vi "Configuration Tool Main.vi"() -> ()   [LabVIEW 2015, in "Configuration Tool.lvlib"]
doc: "This is the main VI for the configuration editor."
uses:
  Configuration Tool.lvlib
  Controls/StateCluster.ctl
  <vilib>/NI/Configuration Framework/Repository/NISE_CEF_Repository.lvclass
  <vilib>/NI/Configuration Framework/Node/NodeRef.ctl
  <vilib>/NI/Configuration Framework/Node/NISE_CEF_Node.lvclass
  <vilib>/NI/Configuration Framework/Node/StandardEvents.ctl
  <vilib>/NI/Configuration Framework/Node/UserEventRef.ctl
  <vilib>/NI/Configuration Framework/Controls/EventCluster.ctl
  <vilib>/NI/Configuration Framework/Node/NodeChangeEvent.ctl
  <vilib>/NI/Configuration Framework/Node/CacheState.ctl
  <vilib>/NI/Configuration Framework/Node/RefreshUIEvent.ctl
  <vilib>/NI/Configuration Framework/Node/StopEvent.ctl
  <vilib>/NI/Configuration Framework/glyph manager/glyph manager.ctl
  <vilib>/picture/picture.llb/imagedata.ctl
  Controls/AddMessage.ctl
  Controls/MoveMessage.ctl
  <vilib>/Utility/error.llb/DialogType.ctl
  Classes/Custom Device/CustomDevice.lvclass
  Classes/CustomDeviceRepo/CustomDeviceRepo.lvclass
  <vilib>/Utility/sysdir.llb/System Directory Type.ctl
  <vilib>/NI/AMC/Read Termination Message.vi
  <vilib>/NI/AMC/Create Single Message.vi
  <vilib>/NI/AMC/Update Message Routing Info.vi
  subVI/Global Settings.vi
  <vilib>/NI/AMC/Globals.vi
  <vilib>/NI/AMC/Send Message.vi
  <vilib>/NI/AMC/AMC.lvlib
  <vilib>/NI/Configuration Framework/NISE_CEF_TreeControl.lvlib
  <vilib>/NI/Configuration Framework/glyph manager/glyph manager.lvlib
panel:
  in  "Target Project":string(combo)
  in  "VeriStand Version":enum16{"2013", "2014", "2015", "2016"}(ring)=enum."2015"
  in  "View":string(tree)
  in  "Exit":bool
  # "Custom Device XML Editor"
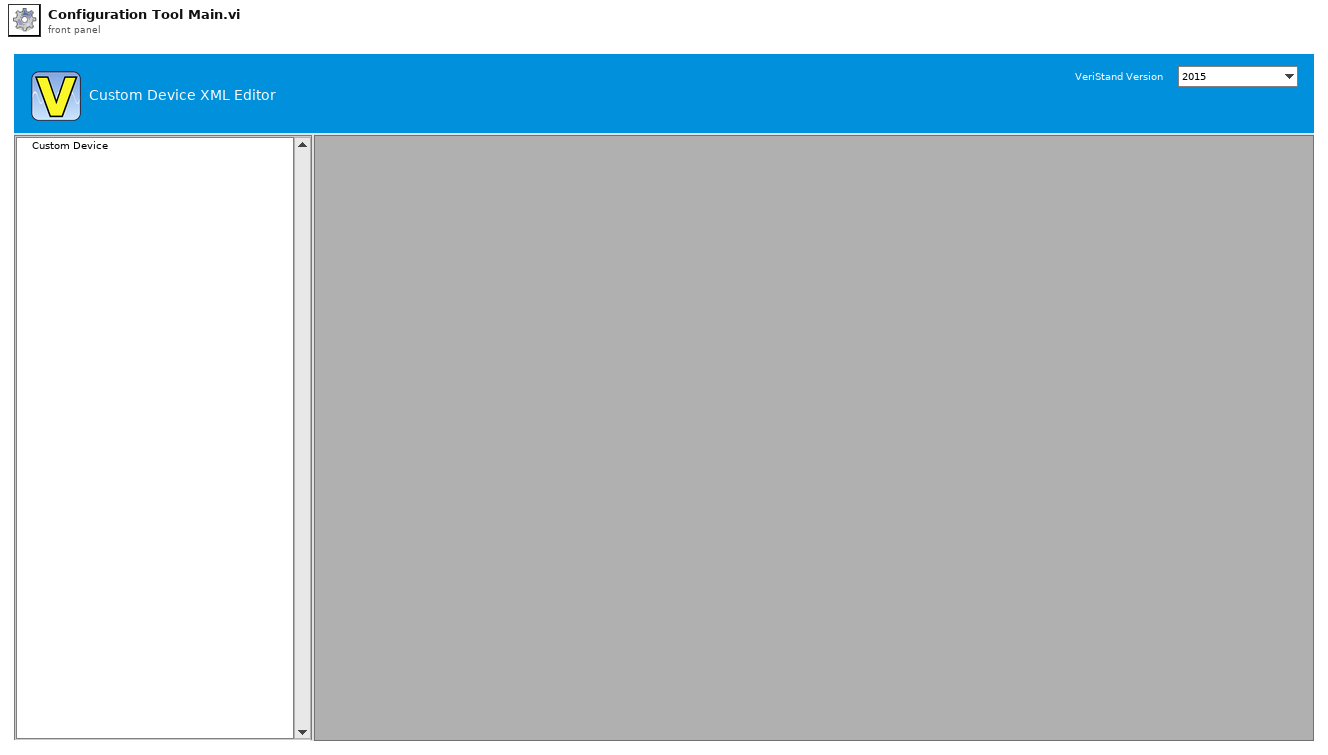
[diagram p1: front panel]
types:
  T1 = typedef "Configuration Tool.lvlib/StateCluster.ctl" = cluster{"repository":refnum<class "NISE_CEF_Repository.lvclass">, "root":T2, "unsaved changes":bool, "current path":path, "standard events":T3, "classes path":path, "glyph manager":T9}
  T2 = typedef "NISE_CEF_Node.lvclass/NodeRef.ctl" = refnum<data-value>
  T3 = typedef "NISE_CEF_Node.lvclass/StandardEvents.ctl" = cluster{"user event":T4, "node change":T5, "cache state":T6, "refresh UI":T7, "stop event":T8}
  T4 = typedef "NISE_CEF_Node.lvclass/UserEventRef.ctl" = refnum<user-event>
  T5 = typedef "NISE_CEF_Node.lvclass/NodeChangeEvent.ctl" = refnum<user-event>
  T6 = typedef "NISE_CEF_Node.lvclass/CacheState.ctl" = refnum<user-event>
  T7 = typedef "NISE_CEF_Node.lvclass/RefreshUIEvent.ctl" = refnum<user-event>
  T8 = typedef "NISE_CEF_Node.lvclass/StopEvent.ctl" = refnum<user-event>
  T9 = typedef "glyph manager.lvlib/glyph manager.ctl" = cluster{"search paths":path[], "glyph map":variant, "base glyphs":T10[], "desired overlays":string[]}
  T10 = typedef "imagedata.ctl" = cluster{"image type":i32, "image depth":i32, "image":u8[], "mask":u8[], "colors":u32[], "Rectangle":cluster{"left":i16, "top":i16, "right":i16, "bottom":i16}}
  T11 = cluster{"Names":string[], "Project refs":refnum<vi>[]}
  T12 = typedef "AMC.lvlib/Message Queue.ctl" = refnum<queue>
  T13 = typedef "Configuration Tool.lvlib/AddMessage.ctl" = cluster{"node type":string, "to add to":string}
  T14 = typedef "Configuration Tool.lvlib/MoveMessage.ctl" = cluster{"node ref":T2, "new parent":T2}
  T15 = typedef "Configuration Tool.lvlib/FilePaths.ctl" = cluster{"glyphs":path, "classes":path}
  T16 = typedef "DialogType.ctl" = u16
  T17 = typedef "System Directory Type.ctl" = i32
  T18 = typedef "NISE_CEF_Node.lvclass/Summary.ctl" = cluster{"ID":string, "parent ID":string, "node type":string, "text":string, "additional text":string, "glyph":string, "depth":i32, "glyph overlay":string}
  T19 = typedef "LVPoint32TypeDef.ctl" = cluster{"Horizontal":i32, "Vertical":i32}
  T20 = cluster{"data name":string, "drag data":variant}[]
  T21 = typedef "NISE_CEF_Node.lvclass/NodeMenuOptions.ctl" = cluster{"removable":bool, "movable":bool, "duplicate":bool}
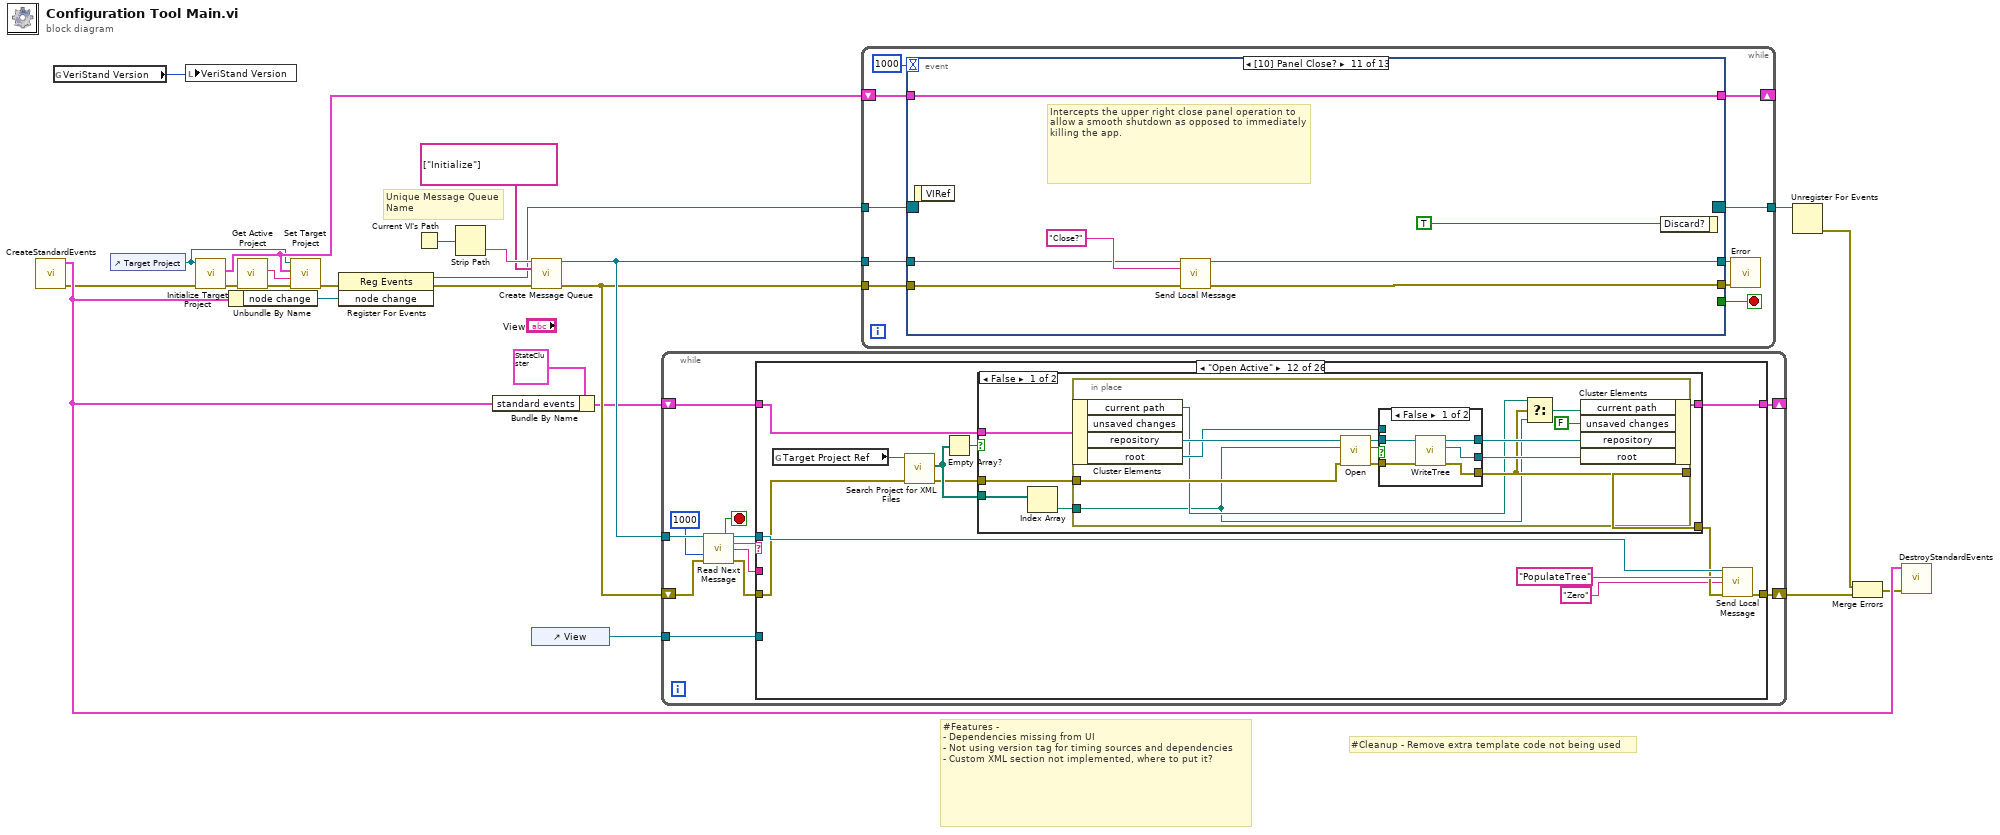
[diagram p0: block diagram]
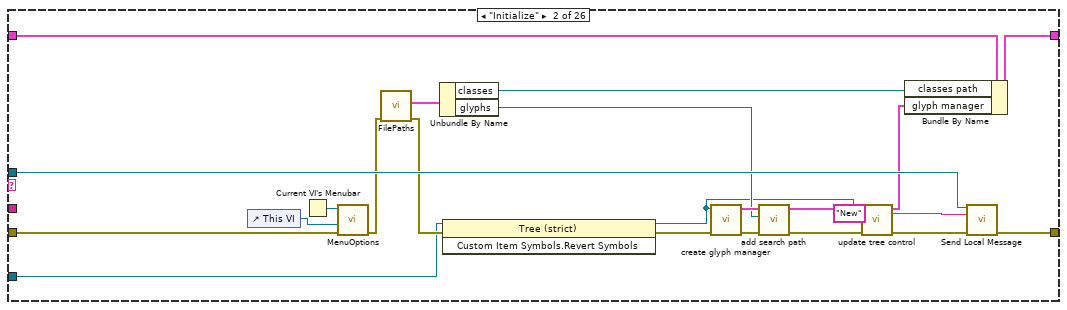
[diagram p3: hidden frame]
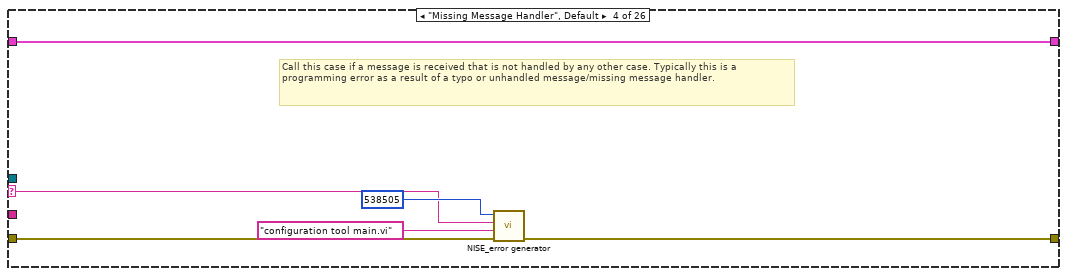
[diagram p5: hidden frame]
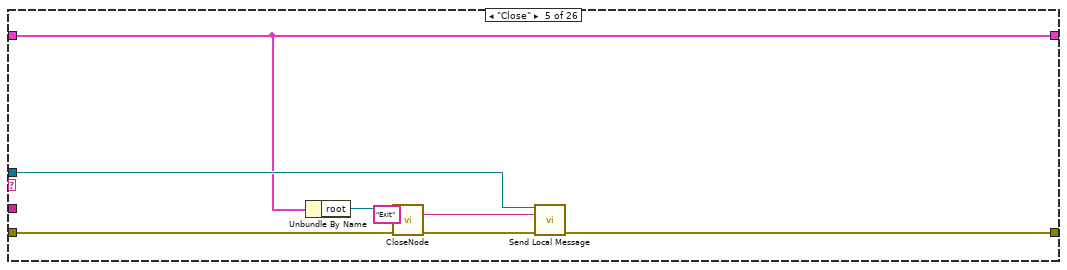
[diagram p6: hidden frame]
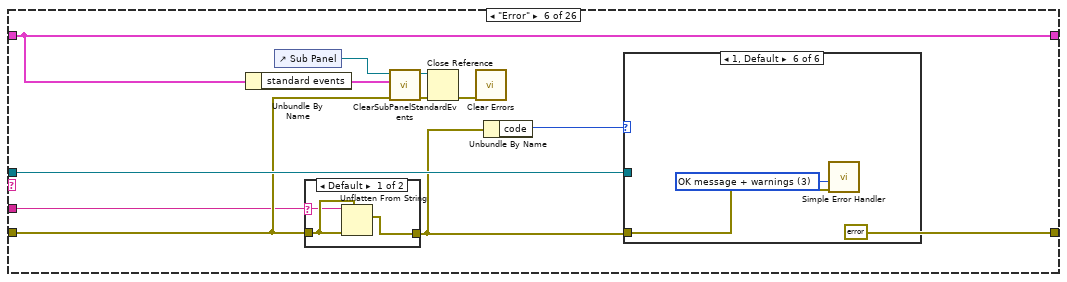
[diagram p7: hidden frame]
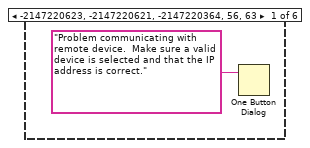
[diagram p9: hidden frame]
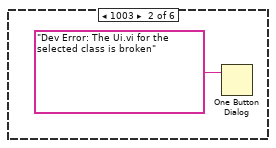
[diagram p10: hidden frame]
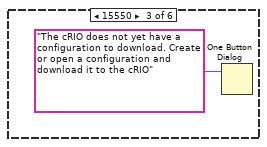
[diagram p11: hidden frame]
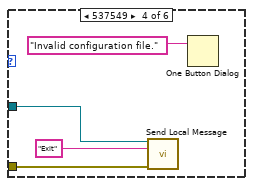
[diagram p12: hidden frame]
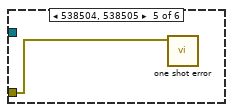
[diagram p13: hidden frame]
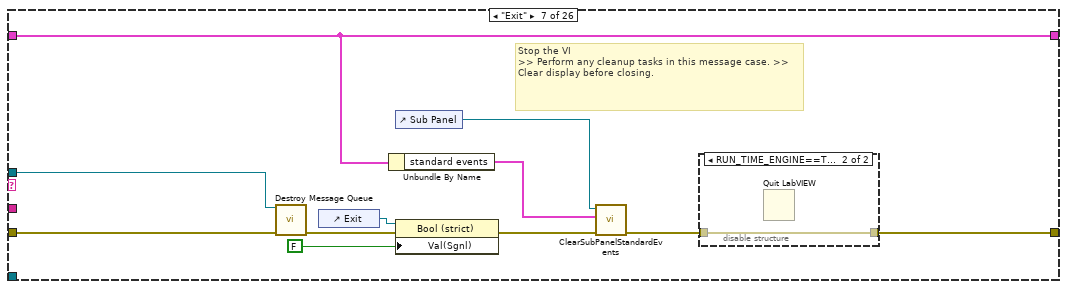
[diagram p14: hidden frame]
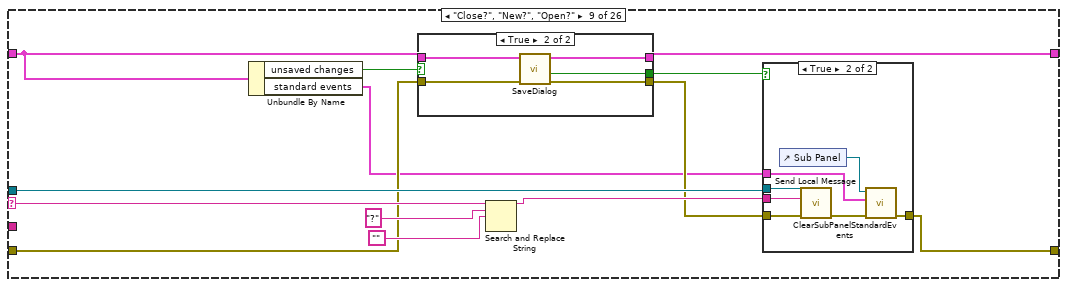
[diagram p17: hidden frame]
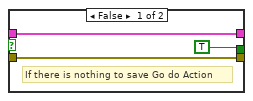
[diagram p18: hidden frame]
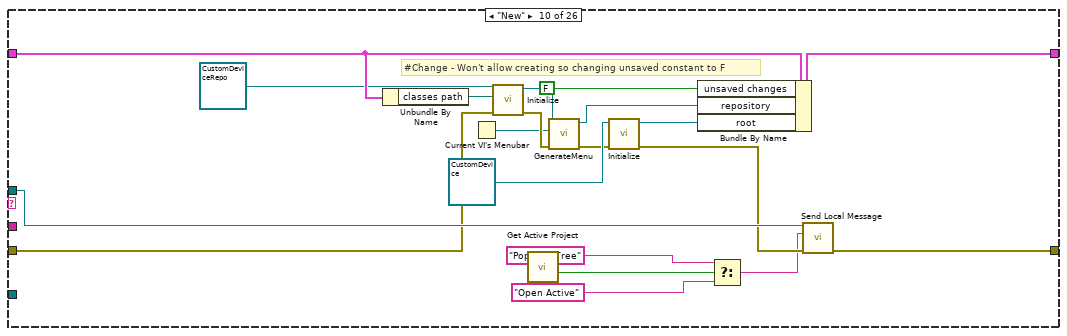
[diagram p20: hidden frame]
diagram:
  # "#Cleanup - Remove extra template code not being used"
  # "#Features - \n- Dependencies missing from UI\n- Not using version tag for timing sources and dependencies\n- Custom XML section not implemented, where to put it?"
  # "Unique Message Queue Name"
  n1 = call <vilib>:"CreateStandardEvents.vi"() -> ("error out"=w2:errorcluster, "standard events"=w14:T3)  [unwired: 10 in]
  n2 = global read "Global Settings.vi" "VeriStand Version"() -> (w8:enum16{"2013", "2014", "2015", "2016"})
  n3 = control-ref of="Target Project"() -> (w3:refnum<vi>)
  n4 = local write "VeriStand Version"(w8) -> ()
  n5 = call "Initialize Target Project.vi"("error in (no error)"=w2, "ComboBox in"=w3) -> ("error out"=w7:errorcluster, "Projects"=w5:T11)  [unwired: 8 in]
  n6 = Unbundle By Name(w14) -> ("node change"=w19:T5)
  n7 = call "Get Active Project.vi"("error in (no error)"=w7) -> ("error out"=w6:errorcluster, "Name"=w4:string)  [unwired: 7 in, 2 out]
  n8 = call "Set Target Project.vi"("error in (no error)"=w6, "Target Project"=w4, "Projects"=w5, "ComboBox Ref"=w3) -> ("error out"=w1:errorcluster)  [unwired: 7 in]
  n9 = register-events(error in=w1, w19) -> (reference out=w13:refnum<event-registration>, error out=w18:errorcluster)  [unwired: 1 in]
  n10 = Current VI's Path() -> (path=w23:path)
  n11 = Strip Path(path=w23) -> (name=w24:string)  [unwired: 1 out]
  n12 = Bundle By Name(cluster=T1 {"repository"=refnum, "root"=refnum, "unsaved changes"=FALSE, "current path"=path "", "standard events"={"user event"=refnum, "node change"=refnum, "cache state"=refnum, "refresh UI"=refnum, "stop event"=refnum}, "classes path"=path "", "glyph manager"={"search paths"=[], "glyph map"=variant, "base glyphs"=[], "desired overlays"=[]}}, "standard events"=w14) -> (w16:T1)
  n13 = call <vilib>:"Create Message Queue.vi"("message queue name"=w24, "initial message names"=string[] ["Initialize"], "error in"=w18) -> ("message queue out"=w21:T12, "error out"=w20:errorcluster)  [unwired: 11 in]
  n14 = control-ref of="View"() -> (w12:refnum<vi>)
  n15 = while "Message Processor" {
    shift-right: [w32] -> w15
    shift-left: w20 -> [w31]
    tunnel: w21 -> [w30]
    shift-right: [w28] -> _
    shift-left: w16 -> [w27]
    tunnel: w12 -> [w25]
    stop <- w36 stop-if-true
    n16 = call <vilib>:"Read Next Message.vi"("message queue in"=w30, "timeout (1 ms)"=1000, "error in"=w31) -> ("exit process?"=w36:bool, "message queue out"=w26:T12, "message name"=w35:string, "message value"=w34:string, "error out"=w33:errorcluster)  [unwired: 5 in, 3 out]
    n17 = case shown="\"Open Active\"" w35 {
      selector: w35 -> [_ _ _ w64 _ _ _ _ w125 _ _ _ _ _ _ _ _ _ w382 _ _ _ _ _ _ _]
      tunnel: w34 -> [_ _ _ _ _ w77 _ _ _ _ _ _ _ _ w291 _ w343 w360 w380 w432 w456 w467 _ w516 w536 w543]
      tunnel: w33 -> [w38 w60 w62 w67 w70 w80 w112 w116 w118 w159 w179 w218 w261 w283 w298 w311 w336 w359 w385 w434 w455 w484 w506 w515 w534 w544]
      tunnel: [w38 w56 w62 w65 w74 errorcluster {"status"=FALSE, "code"=0, "source"=""} ("error out") w104 w116 w129 w165 w175 w223 w258 w285 w295 w311 w315 w363 w388 w436 w452 w471 w502 w512 w529 w542] -> w32
      tunnel: [w37 w52 w61 w68 w72 w84 w103 w115 w120 w163 w180 w227 w264 w284 w292 w310 w331 w356 w389 w435 w457 w477 w505 w510 w537 w539] -> w28
      tunnel: w27 -> [w37 w53 w61 w68 w72 w84 w103 w115 w121 w161 w181 w228 w263 w282 w293 w310 w334 w357 w389 w427 w457 w486 w505 w510 w537 w545]
      tunnel: w26 -> [_ w55 _ _ w73 w87 w111 _ w128 w164 w177 w225 _ _ w294 _ w312 _ w383 _ _ _ _ w511 w528 w541]
      tunnel: w25 -> [_ w41 _ _ _ _ _ _ _ _ _ _ _ _ _ _ w332 w352 w377 w429 w450 w473 _ _ _ _]
      frame "------------Generic Operations------------" {
        # "Dummy case to add a seperation in the Case Structure menu"
      }
      frame "Initialize" {
        n18 = control-ref of="This VI"() -> (w59:refnum<vi>)
        n19 = Current VI's Menubar() -> (w58:refnum<k9>)
        n20 = call "MenuOptions.vi"("error in"=w60, "VI ref"=w59, "menu ref in"=w58) -> ("error out"=w51:errorcluster)  [unwired: 7 in, 1 out]
        n21 = call "FilePaths.vi"("error in"=w51) -> ("error out"=w44:errorcluster, "paths"=w54:T15)  [unwired: 9 in]
        n22 = Unbundle By Name(w54) -> ("classes"=w50:path, "glyphs"=w46:path)
        n23 = invoke class="Tree (strict)" method="Custom Item Symbols.Revert Symbols"(reference=w41, error in=w44) -> (reference out=w42:refnum<vi>, error out=w43:errorcluster)  [unwired: 1 in, 1 out]
        n24 = call <vilib>:"create glyph manager.vi"("error in"=w43, "tree ref (for default symbols)"=w42) -> ("error out"=w49:errorcluster, "glyph manager"=w48:T9)  [unwired: 8 in]
        n25 = call <vilib>:"add search path.vi"("error in"=w49, "search path"=w46, "glyph manager in"=w48) -> ("error out"=w40:errorcluster, "glyph manager out"=w39:T9)  [unwired: 7 in]
        n26 = call <vilib>:"update tree control.vi"("error in"=w40, "tree reference"=w42, "glyph manager in"=w39) -> ("error out"=w47:errorcluster, "glyph manager out"=w45:T9)  [unwired: 7 in]
        n27 = Bundle By Name(cluster=w53, "classes path"=w50, "glyph manager"=w45) -> (w52:T1)
        n28 = call <vilib>:"Send Local Message.vi"("message queue in"=w55, "message name"="New" ("Message Name"), "error in"=w47) -> ("error out"=w56:errorcluster)  [unwired: 10 in, 2 out]
      }
      frame "", "Idle" {
      }
      frame "Missing Message Handler", Default {
        # "Call this case if a message is received that is not handled by any other case. Typically this is a programming error as a result of a typo or unhandled message/missing message handler."
        n29 = call <vilib>:"NISE_error generator.vi"("error in"=w67, "source"="configuration tool main.vi", "append error message"=w64, "error code (0)"=538505) -> ("error out"=w65:errorcluster)  [unwired: 5 in]
      }
      frame "Close" {
        n30 = Unbundle By Name(w72) -> ("root"=w71:T2)
        n31 = call <vilib>:"CloseNode.vi"("error in"=w70, "node ref"=w71) -> ("error out"=w69:errorcluster)  [unwired: 9 in]
        n32 = call <vilib>:"Send Local Message.vi"("message queue in"=w73, "message name"="Exit", "error in"=w69) -> ("error out"=w74:errorcluster)  [unwired: 10 in, 2 out]
      }
      frame "Error" {
        n33 = Unbundle By Name(w84) -> ("standard events"=w76:T3)
        n34 = control-ref of="Sub Panel"() -> (w83:refnum<vi>)
        n35 = case shown="Default" w77 {
          selector: w77 -> [w89 _]
          tunnel: w80 -> [w90 w91]
          tunnel: [w88 w91] -> w79
          frame Default {
            n36 = Unflatten From String(type=w90, binary string=w89, error in (no error)=w90) -> (value=w88:errorcluster)  [unwired: 2 in, 2 out]
          }
          frame "" {
          }
        }
        n37 = call <vilib>:"ClearSubPanelStandardEvents.vi"("error in"=w80, "standard events"=w76, "sub panel ref in"=w83) -> ("error out"=w82:errorcluster, "sub panel ref out"=w81:refnum<vi>)  [unwired: 7 in]
        n38 = Close Reference(reference=w81, error in (no error)=w82) -> (error out=w78:errorcluster)
        n39 = call <vilib>:"Clear Errors.vi"("error in (no error)"=w78) -> ()  [unwired: 5 in, 2 out]
        n40 = Unbundle By Name(w79) -> ("code"=w85:i32)
        n41 = case shown="1, Default" w85 {
          tunnel: w87 -> [_ _ _ w97 _ _]
          tunnel: w79 -> [_ _ _ w96 w99 w101]
          frame -2147220623, -2147220621, -2147220364, 56, 63 {
            n42 = One Button Dialog(message="Problem communicating with remote device.  Make sure a valid device is selected and that the IP address is correct.") -> ()  [unwired: 1 in, 1 out]
          }
          frame 1003 {
            n43 = One Button Dialog(message="Dev Error: The Ui.vi for the selected class is broken") -> ()  [unwired: 1 in, 1 out]
          }
          frame 15550 {
            n44 = One Button Dialog(message="The cRIO does not yet have a configuration to download. Create or open a configuration and download it to the cRIO") -> ()  [unwired: 1 in, 1 out]
          }
          frame 537549 {
            n45 = call <vilib>:"Send Local Message.vi"("message queue in"=w97, "message name"="Exit", "error in"=w96) -> ()  [unwired: 10 in, 3 out]
            n46 = One Button Dialog(message="Invalid configuration file.") -> ()  [unwired: 1 in, 1 out]
          }
          frame 538504, 538505 {
            n47 = call <vilib>:"one shot error.vi"("error in"=w99) -> ()  [unwired: 11 in]
          }
          frame 1, Default {
            w100 = T16 3 items=["no dialog", "OK message", "continue or stop message", "OK message + warnings", "continue/stop + warnings"] ("type of dialog (OK msg:1)")
            n48 = call <vilib>:"Simple Error Handler.vi"("type of dialog (OK msg:1)"=w100, "error in (no error)"=w101) -> ()  [unwired: 8 out]
          }
        }
      }
      frame "Exit" {
        # "Stop the VI                                                                             >> Perform any cleanup tasks in this message case. >> Clear display before closing."
        n49 = call <vilib>:"Destroy Message Queue.vi"("message queue in"=w111, "error in"=w112) -> ("error out"=w108:errorcluster)  [unwired: 11 in, 2 out]
        n50 = control-ref of="Exit"() -> (w110:refnum<vi>)
        n51 = Unbundle By Name(w103) -> ("standard events"=w102:T3)
        n52 = control-ref of="Sub Panel"() -> (w107:refnum<vi>)
        n53 = property class="Bool (strict)"(reference=w110, error in=w108, "Val(Sgnl)"=FALSE ("Exit")) -> (error out=w106:errorcluster)  [unwired: 1 out]
        n54 = call <vilib>:"ClearSubPanelStandardEvents.vi"("error in"=w106, "standard events"=w102, "sub panel ref in"=w107) -> ("error out"=w105:errorcluster)  [unwired: 7 in, 1 out]
        n55 = disable-structure shown="RUN_TIME_ENGINE==True" {
          disable-tunnel: [w113 w114] -> w104
          disable-tunnel: w105 -> [w113 w114]
          frame condition #0 (active) {
          }
          frame condition #1 {
            n56 = Quit LabVIEW() -> ()  [unwired: 1 in]
          }
        }
      }
      frame "------------Menu Operations--------------" {
        # "Dummy case to add a seperation in the Case Structure menu"
      }
      frame "Close?", "New?", "Open?" {
        n57 = Unbundle By Name(w121) -> ("unsaved changes"=w123:bool, "standard events"=w117:T3)
        n58 = case shown="True" w123 {
          tunnel: [TRUE ("SaveFlag") w137] -> w122
          tunnel: w121 -> [w131 w136]
          tunnel: [w131 w135] -> w120
          tunnel: w118 -> [w130 w134]
          tunnel: [w130 w133] -> w119
          frame False {
            # "If there is nothing to save Go do Action"
          }
          frame True {
            n59 = call "SaveDialog.vi"("error in"=w134, "state in"=w136) -> ("error out"=w133:errorcluster, "new"=w137:bool, "state out"=w135:T1)  [unwired: 7 in]
          }
        }
        n60 = Search and Replace String(input string=w125, search string="?", replace string="") -> (result string=w124:string)  [unwired: 5 in, 3 out]
        n61 = case shown="True" w122 {
          tunnel: w119 -> [w138 w145]
          tunnel: [w138 w141] -> w129
          tunnel: w128 -> [_ w144]
          tunnel: w124 -> [_ w143]
          tunnel: w117 -> [_ w139]
          frame False {
          }
          frame True {
            n62 = control-ref of="Sub Panel"() -> (w140:refnum<vi>)
            n63 = call <vilib>:"Send Local Message.vi"("message queue in"=w144, "message name"=w143, "error in"=w145) -> ("error out"=w142:errorcluster)  [unwired: 10 in, 2 out]
            n64 = call <vilib>:"ClearSubPanelStandardEvents.vi"("error in"=w142, "standard events"=w139, "sub panel ref in"=w140) -> ("error out"=w141:errorcluster)  [unwired: 7 in, 1 out]
          }
        }
      }
      frame "New" {
        # "#Change - Won't allow creating so changing unsaved constant to F"
        n65 = Unbundle By Name(w161) -> ("classes path"=w160:path)
        n66 = Current VI's Menubar() -> (w155:refnum<k9>)
        n67 = call-dynamic "Initialize.vi"("error in"=w159, "path"=w160, "repository in"=refnum<class "CustomDeviceRepo.lvclass"> refnum ("CustomDeviceRepo.lvclass")) -> ("error out"=w158:errorcluster, "repository out"=w157:refnum<class "CustomDeviceRepo.lvclass">)  [unwired: 7 in]
        n68 = call "Get Active Project.vi"() -> ("No Active Project?"=w149:bool)  [unwired: 8 in, 3 out]
        n69 = call-dynamic "GenerateMenu.vi"("error in"=w158, "menu ref in"=w155, "NISE_CEF_Repository in"=w157) -> ("error out"=w152:errorcluster, "NISE_CEF_Repository out"=w156:refnum<class "CustomDeviceRepo.lvclass">)  [unwired: 6 in, 1 out]
        n70 = call-dynamic "Initialize.vi"("error in"=w152, "node in"=refnum<class "CustomDevice.lvclass"> refnum ("CustomDevice.lvclass")) -> ("error out"=w151:errorcluster, "data value reference"=w154:T2)  [unwired: 7 in, 1 out]
        n71 = Bundle By Name(cluster=w161, "unsaved changes"=FALSE ("SaveFlag"), "repository"=w156, "root"=w154) -> (w163:T1)
        n72 = Select(t="PopulateTree", s=w149, f="Open Active") -> (s? t:f=w146:string)
        n73 = call <vilib>:"Send Local Message.vi"("message queue in"=w164, "message name"=w146, "error in"=w151) -> ("error out"=w165:errorcluster)  [unwired: 10 in, 2 out]
      }
      frame "Open" {
        w174 = T17 6 items=["User Home"=0, "User Desktop"=1, "User Documents"=2, "User Application Data"=3, "User Preferences"=4, "User Temporary"=5, "Public Documents"=6, "Public Application Data"=7, "Public Preferences"=8, "Public Cache"=13, "System Core Libraries"=9, "System Installed Libraries"=10, "Application Files"=11, "Boot Volume Root"=12] ("system directory type")
        n74 = global read "Global Settings.vi" "VeriStand Version"() -> (w167:enum16{"2013", "2014", "2015", "2016"})
        n75 = Format Into String(w167) -> (resulting string=w166:string)  [unwired: 3 in, 1 out]
        n76 = Search and Replace String(input string="National Instruments\\NI VeriStand XXXX\\Custom Devices", search string="XXXX", replace string=w166) -> (result string=w170:string)  [unwired: 5 in, 3 out]
        n77 = call <vilib>:"Get System Directory.vi"("system directory type"=w174) -> ("system directory"=w171:path)  [unwired: 10 in]
        n78 = Build Path(base path=w171, name or relative path=w170) -> (appended path=w169:path)
        n79 = in-place {
          in-place-border: w179 -> [w187]
          in-place-border: [w186] -> w176
          in-place-border: w169 -> [w182]
          n80 = in-place-cluster #1(w181) -> ("current path"=w184:path, "repository"=w195:refnum<class "NISE_CEF_Repository.lvclass">, "root"=w191:T2)  [unwired: 1 out]
          n81 = call "FileDialog.vi"("error in"=w187, "start path"=w182) -> ("error out"=w188:errorcluster, "cancelled"=w189:bool, "selected path"=w185:path)  [unwired: 7 in]
          n82 = Compound Arithmetic op=OR(invert w189) -> (w190:bool)
          n83 = case shown="True" w190 {
            tunnel: w195 -> [w196 w208]
            tunnel: [w196 w206] -> w193
            tunnel: [w197 w204] -> w186
            tunnel: [w198 w203] -> w192
            tunnel: w185 -> [_ w201]
            tunnel: w188 -> [w197 w200]
            tunnel: w191 -> [w198 w199]
            frame False {
            }
            frame True {
              n84 = call-dynamic "Open.vi"("error in"=w200, "file path"=w201, "repository in"=w208) -> ("error out"=w205:errorcluster, "invalid?"=w202:bool, "repository out"=w207:refnum<class "NISE_CEF_Repository.lvclass">)  [unwired: 6 in]
              n85 = case shown="False" w202 {
                tunnel: w207 -> [w213 w216]
                tunnel: [w212 w216] -> w206
                tunnel: w205 -> [w211 w215]
                tunnel: [w210 w215] -> w204
                tunnel: [w209 w214] -> w203
                tunnel: w199 -> [_ w214]
                frame False {
                  n86 = call-dynamic "WriteTree.vi"("error in"=w211, "repository in"=w213) -> ("error out"=w210:errorcluster, "root"=w209:T2, "repository out"=w212:refnum<class "NISE_CEF_Repository.lvclass">)  [unwired: 7 in]
                }
                frame True {
                }
              }
            }
          }
          n87 = Select(t=w184, s=w186, f=w185) -> (s? t:f=w183:path)
          n88 = in-place-cluster #1("current path"=w183, "unsaved changes"=FALSE ("SaveFlag"), "repository"=w193, "root"=w192) -> (w180:T1)
        }
        n89 = call <vilib>:"Send Local Message.vi"("message queue in"=w177, "message name"="PopulateTree", "message value"="Zero", "error in"=w176) -> ("error out"=w175:errorcluster)  [unwired: 9 in, 2 out]
      }
      frame "Open Active" {
        n90 = global read "Global Settings.vi" "Target Project Ref"() -> (w221:refnum<vi>)
        n91 = call "Search Project for XML Files.vi"("error in (no error)"=w218, "project reference"=w221) -> ("error out"=w217:errorcluster, "xml files found"=w220:path[])  [unwired: 8 in]
        n92 = Empty Array?(array=w220) -> (empty?=w219:bool)
        n93 = case shown="False" w219 {
          tunnel: w228 -> [w234 w257]
          tunnel: [w233 w257] -> w227
          tunnel: w217 -> [w232 w256]
          tunnel: [w231 w256] -> w224
          tunnel: w220 -> [w229 _]
          frame False {
            n94 = Index Array(array=w229) -> (element=w230:path)  [unwired: 1 in]
            n95 = in-place {
              in-place-border: w232 -> [w242]
              in-place-border: [w241] -> w231
              in-place-border: w230 -> [w235]
              n96 = in-place-cluster #2(w234) -> ("current path"=w240:path, "repository"=w247:refnum<class "NISE_CEF_Repository.lvclass">, "root"=w243:T2)  [unwired: 1 out]
              n97 = call-dynamic "Open.vi"("error in"=w242, "file path"=w235, "repository in"=w247) -> ("error out"=w237:errorcluster, "invalid?"=w236:bool, "repository out"=w238:refnum<class "NISE_CEF_Repository.lvclass">)  [unwired: 6 in]
              n98 = case shown="False" w236 {
                tunnel: w238 -> [w252 w255]
                tunnel: [w251 w255] -> w245
                tunnel: w237 -> [w250 w254]
                tunnel: [w249 w254] -> w241
                tunnel: [w248 w253] -> w244
                tunnel: w243 -> [_ w253]
                frame False {
                  n99 = call-dynamic "WriteTree.vi"("error in"=w250, "repository in"=w252) -> ("error out"=w249:errorcluster, "root"=w248:T2, "repository out"=w251:refnum<class "NISE_CEF_Repository.lvclass">)  [unwired: 7 in]
                }
                frame True {
                }
              }
              n100 = Select(t=w240, s=w241, f=w235) -> (s? t:f=w239:path)
              n101 = in-place-cluster #2("current path"=w239, "unsaved changes"=FALSE ("SaveFlag"), "repository"=w245, "root"=w244) -> (w233:T1)
            }
          }
          frame True {
          }
        }
        n102 = call <vilib>:"Send Local Message.vi"("message queue in"=w225, "message name"="PopulateTree", "message value"="Zero", "error in"=w224) -> ("error out"=w223:errorcluster)  [unwired: 9 in, 2 out]
      }
      frame "Save" {
        n103 = in-place {
          in-place-border: w261 -> [w268]
          in-place-border: [w267] -> w260
          in-place-border: [w265] -> w259
          n104 = in-place-cluster #3(w263) -> ("current path"=w266:path, "root"=w269:T2, "repository"=w271:refnum<class "NISE_CEF_Repository.lvclass">)
          n105 = Empty String/Path?(string/path=w266) -> (empty?=w265:bool)
          n106 = call-dynamic "ReadTree.vi"("error in"=w268, "root"=w269, "repository in"=w271) -> ("error out"=w267:errorcluster, "repository out"=w270:refnum<class "NISE_CEF_Repository.lvclass">)  [unwired: 7 in]
          n107 = in-place-cluster #3("current path"=w266, "root"=w269, "repository"=w270) -> (w262:T1)
        }
        n108 = case shown="False" w259 {
          tunnel: w262 -> [w275 w277]
          tunnel: [w274 w276] -> w264
          tunnel: [w273 w278] -> w258
          tunnel: w260 -> [w272 w279]
          frame False {
            n109 = call "Save.vi"("error in"=w272, "state in"=w275) -> ("error out"=w273:errorcluster, "state out"=w274:T1)  [unwired: 8 in]
          }
          frame True {
            # "Empty path use Dialog"
            n110 = call "SaveAs.vi"("error in"=w279, "state in"=w277) -> ("error out"=w278:errorcluster, "state out"=w276:T1)  [unwired: 7 in, 1 out]
          }
        }
      }
      frame "SaveAs" {
        n111 = in-place {
          in-place-border: w283 -> [w287]
          in-place-border: [w286] -> w281
          n112 = in-place-cluster #4(w282) -> ("root"=w288:T2, "repository"=w290:refnum<class "NISE_CEF_Repository.lvclass">)
          n113 = call-dynamic "ReadTree.vi"("error in"=w287, "root"=w288, "repository in"=w290) -> ("error out"=w286:errorcluster, "repository out"=w289:refnum<class "NISE_CEF_Repository.lvclass">)  [unwired: 7 in]
          n114 = in-place-cluster #4("root"=w288, "repository"=w289) -> (w280:T1)
        }
        n115 = call "SaveAs.vi"("error in"=w281, "state in"=w280) -> ("error out"=w285:errorcluster, "state out"=w284:T1)  [unwired: 7 in, 1 out]
      }
      frame "Custom View" {
        n116 = in-place {
          in-place-border: w298 -> [w309]
          in-place-border: [w308] -> w296
          in-place-border: w291 -> [w299]
          n117 = in-place-cluster #5(w293) -> ("repository"=w303:refnum<class "NISE_CEF_Repository.lvclass">, "root"=w302:T2)
          n118 = call-dynamic "ReadTree.vi"("error in"=w309, "root"=w302, "repository in"=w303) -> ("error out"=w306:errorcluster, "repository out"=w305:refnum<class "NISE_CEF_Repository.lvclass">)  [unwired: 7 in]
          n119 = call-dynamic "CustomView.vi"("error in"=w306, "view name"=w299, "repository in"=w305) -> ("error out"=w307:errorcluster, "repository out"=w304:refnum<class "NISE_CEF_Repository.lvclass">)  [unwired: 7 in]
          n120 = call-dynamic "WriteTree.vi"("error in"=w307, "repository in"=w304) -> ("error out"=w308:errorcluster, "root"=w300:T2, "repository out"=w301:refnum<class "NISE_CEF_Repository.lvclass">)  [unwired: 7 in]
          n121 = in-place-cluster #5("repository"=w301, "root"=w300) -> (w292:T1)
        }
        n122 = call <vilib>:"Send Local Message.vi"("message queue in"=w294, "message name"="PopulateTree", "error in"=w296) -> ("error out"=w295:errorcluster)  [unwired: 10 in, 2 out]
      }
      frame "-------TreeControl Operations-----------" {
        # "Dummy case to add a seperation in the Case Structure menu"
      }
      frame "AddNode" {
        # "#Change - Added ability for added nodes\nto then add children"
        # "#Change - Had to make own copy\nof add node since CEF framework\ndoesn't let you pass params to init"
        # "#Change - Look for potential\ndashes for menu items with\nparameterized options"
        n123 = Unflatten From String(type=T13 {"node type"="", "to add to"=""} ("input cluster"), binary string=w343) -> (value=w341:T13)  [unwired: 3 in, 2 out]
        n124 = Unbundle By Name(w341) -> ("to add to"=w339:string, "node type"=w321:string)
        n125 = Match Pattern(string=w321, regular expression="\\-") -> (before substring=w320:string, after substring=w319:string)  [unwired: 1 in, 2 out]
        n126 = in-place {
          in-place-border: w336 -> [w349]
          in-place-border: [w348] -> w335
          in-place-border: w320 -> [w347]
          in-place-border: [w346] -> w333
          n127 = in-place-cluster #6(w334) -> ("repository"=w351:refnum<class "NISE_CEF_Repository.lvclass">)
          n128 = call-dynamic "GetClassPath.vi"("error in"=w349, "class name"=w347, "Repository in"=w351) -> ("error out"=w348:errorcluster, "class path"=w346:path, "Repository out"=w350:refnum<class "NISE_CEF_Repository.lvclass">)  [unwired: 6 in]
          n129 = in-place-cluster #6("repository"=w350) -> (w328:T1)
        }
        n130 = Unbundle By Name(w328) -> ("glyph manager"=w327:T9)
        n131 = call <vilib>:"Get LV Class Default Value.vi"("error in (no error)"=w335, "class path"=w333) -> ("error out"=w344:errorcluster, "object"=w345:refnum<class>)  [unwired: 8 in]
        n132 = To More Specific Class(target class=refnum<class "NISE_CEF_Node.lvclass"> refnum ("Node.lvclass"), reference=w345, error in=w344) -> (specific class reference=w329:refnum<class "NISE_CEF_Node.lvclass">, error out=w330:errorcluster)
        n133 = call-dynamic "AddGlyphtoGManager.vi"("error in"=w330, "glyph manager"=w327, "NISE_CEF_Node in"=w329) -> ("error out"=w325:errorcluster, "glyph manager out"=w326:T9, "NISE_CEF_Node out"=w324:refnum<class "NISE_CEF_Node.lvclass">)  [unwired: 6 in]
        n134 = Match Pattern(string=w319, regular expression="\\-") -> (before substring=w317:string, after substring=w314:string)  [unwired: 1 in, 2 out]
        n135 = call "Modified Framework AddNode.vi"("parameters"=w317, "error in"=w325, "node in"=w324, "parent node ID"=w339) -> ("error out"=w338:errorcluster, "summary"=w337:T18[], "ID of Added Node"=w313:string)  [unwired: 5 in]
        n136 = call <vilib>:"PopulateTreeSumaryWithGlyphManager.vi"("error in"=w338, "glyph manager"=w326, "summary"=w337, "tree ref in"=w332) -> ("error out"=w316:errorcluster, "glyph manager out"=w323:T9)  [unwired: 6 in]
        n137 = Bundle By Name(cluster=w328, "glyph manager"=w323) -> (w331:T1)
        n138 = call "Send Message to Create Child Object.vi"("Error In"=w316, "ID of Node to Add To"=w313, "node type"=w314, "Queue in"=w312) -> ("Error Out"=w315:errorcluster)  [unwired: 6 in, 1 out]
      }
      frame "Duplicate" {
        n139 = call <vilib>:"IDtoNode.vi"("error in"=w359, "ID"=w360) -> ("error out"=w361:errorcluster, "invalid Id"=w358:bool, "node ref"=w362:T2)  [unwired: 7 in]
        n140 = Unbundle By Name(w357) -> ("glyph manager"=w354:T9)
        n141 = case shown="False" w358 {
          tunnel: [w374 w376] -> w363
          tunnel: w362 -> [w373 _]
          tunnel: w361 -> [w370 w376]
          tunnel: w354 -> [w366 w375]
          tunnel: [w365 w375] -> w353
          tunnel: w352 -> [w364 _]
          frame False {
            n142 = call <vilib>:"DuplicateNode.vi"("same parent?"=TRUE ("s"), "error in"=w370, "node ref in"=w373) -> ("error out"=w371:errorcluster, "new node ref"=w372:T2)  [unwired: 7 in]
            n143 = call <vilib>:"Summary.vi"("error in"=w371, "node self ref"=w372) -> ("error out"=w368:errorcluster, "summary"=w367:T18[])  [unwired: 8 in]
            n144 = call <vilib>:"PopulateTreeSumaryWithGlyphManager.vi"("error in"=w368, "glyph manager"=w366, "summary"=w367, "tree ref in"=w364) -> ("error out"=w374:errorcluster, "glyph manager out"=w365:T9)  [unwired: 6 in]
          }
          frame True {
          }
        }
        n145 = Bundle By Name(cluster=w357, "unsaved changes"=TRUE, "glyph manager"=w353) -> (w356:T1)
      }
      frame "CustomMenuAction" {
        n146 = Match Pattern(string=w380, regular expression=":") -> (before substring=w379:string, after substring=w378:string)  [unwired: 1 in, 2 out]
        n147 = call <vilib>:"IDtoNode.vi"("error in"=w385, "ID"=w378) -> ("error out"=w386:errorcluster, "invalid Id"=w384:bool, "node ref"=w387:T2)  [unwired: 7 in]
        n148 = case shown="False" w384 {
          tunnel: [w395 w425] -> w388
          tunnel: w387 -> [w392 _]
          tunnel: w386 -> [w398 w425]
          tunnel: w383 -> [w399 _]
          tunnel: w382 -> [_ _]
          tunnel: w379 -> [w396 _]
          tunnel: w377 -> [w393 _]
          frame False {
            n149 = in-place {
              in-place-border: w399 -> [w423]
              in-place-border: w398 -> [w421]
              in-place-border: [w420] -> w394
              in-place-border: [w419] -> w397
              in-place-border: w396 -> [w418]
              in-place-border: w393 -> [w417]
              in-place-border: [w416] -> w391
              n150 = in-place-dvr #7(w392) -> (w424:refnum<class "NISE_CEF_Node.lvclass">)  [unwired: 1 out]
              n151 = call-dynamic "MenuHandler.vi"("tree control"=w417, "main message queue"=w423, "error in"=w421, "menu string"=w418, "NISE_CEF_Node in"=w424) -> ("error out"=w420:errorcluster, "refresh tree?"=w416:bool, "Unhandled"=w419:bool, "NISE_CEF_Node out"=w422:refnum<class "NISE_CEF_Node.lvclass">)  [unwired: 3 in]
              n152 = in-place-dvr #7(w422) -> (w390:T2)  [unwired: 1 out]
            }
            n153 = case shown="True" w397 {
              tunnel: w396 -> [_ w411]
              tunnel: [w403 w412] -> w395
              tunnel: w394 -> [w401 w413]
              tunnel: w391 -> [w400 _]
              tunnel: w390 -> [w402 _]
              frame False {
                n154 = case shown="True" w400 {
                  tunnel: [w404 w407] -> w403
                  tunnel: w402 -> [_ w406]
                  tunnel: w401 -> [w404 w405]
                  frame False {
                  }
                  frame True {
                    n155 = call <vilib>:"NodetoID.vi"("error in"=w405, "node ref"=w406) -> ("error out"=w409:errorcluster, "ID"=w410:string)  [unwired: 8 in]
                    n156 = call <vilib>:"Send Local Message.vi"("message name"="NodeDataChange", "message value"=w410, "error in"=w409) -> ("error out"=w407:errorcluster)  [unwired: 10 in, 2 out]
                  }
                }
              }
              frame True {
                n157 = call <vilib>:"NISE_error generator.vi"("error in"=w413, "source"="configuration tool main.vi", "append error message"=w411, "error code (0)"=538506) -> ("error out"=w412:errorcluster)  [unwired: 5 in]
              }
            }
          }
          frame True {
          }
        }
      }
      frame "RefreshNode" {
        # "Refreshes the node in the Tree, Sets the save flag to true. This case can be called from the UIs of the nodes"
        n158 = Unbundle By Name(w427) -> ("glyph manager"=w426:T9)
        n159 = call <vilib>:"IDtoNode.vi"("error in"=w434, "ID"=w432) -> ("error out"=w433:errorcluster, "invalid Id"=w430:bool, "node ref"=w431:T2)  [unwired: 7 in]
        n160 = case shown="False" w430 {
          tunnel: [w446 w449] -> w436
          tunnel: w433 -> [w442 w449]
          tunnel: w431 -> [w441 _]
          tunnel: w429 -> [w440 _]
          tunnel: [w439 w448] -> w428
          tunnel: w426 -> [w437 w448]
          frame False {
            n161 = call <vilib>:"SummaryWithGlyphManager.vi"("error in"=w442, "glyph manager"=w437, "node self ref"=w441) -> ("error out"=w444:errorcluster, "glyph manager out"=w438:T9, "summary"=w443:T18[])  [unwired: 6 in]
            n162 = call <vilib>:"RefreshSubTreeWithGlyphManager.vi"("error in"=w444, "glyph manager"=w438, "node information"=w443, "tree ref in"=w440) -> ("error out"=w447:errorcluster, "glyph manager out"=w439:T9, "tree ref out"=w445:refnum<vi>)  [unwired: 5 in]
            n163 = Close Reference(reference=w445, error in (no error)=w447) -> (error out=w446:errorcluster)
          }
          frame True {
          }
        }
        n164 = Bundle By Name(cluster=w427, "glyph manager"=w428) -> (w435:T1)
      }
      frame "RemoveNode" {
        n165 = call <vilib>:"IDtoNode.vi"("error in"=w455, "ID"=w456) -> ("error out"=w454:errorcluster, "invalid Id"=w451:bool, "node ref"=w453:T2)  [unwired: 7 in]
        n166 = case shown="False" w451 {
          tunnel: w454 -> [w463 w464]
          tunnel: w453 -> [w462 _]
          tunnel: [w459 w464] -> w452
          tunnel: w450 -> [w458 _]
          frame False {
            n167 = call <vilib>:"RemoveNode.vi"("error in"=w463, "node"=w462) -> ("error out"=w460:errorcluster, "node ID"=w461:string)  [unwired: 8 in]
            n168 = call <vilib>:"ClearTreeNode.vi"("error in"=w460, "tag"=w461, "tree reference"=w458) -> ("error out"=w459:errorcluster)  [unwired: 8 in]
          }
          frame True {
          }
        }
      }
      frame "PopulateTree" {
        n169 = Unbundle By Name(w486) -> ("standard events"=w478:T3, "glyph manager"=w475:T9, "root"=w482:T2)
        n170 = String Length(string=w467) -> (length=w466:i32)
        n171 = Greater Than 0?(x=w466) -> (x > 0?=w465:bool)
        n172 = call <vilib>:"SummaryWithGlyphManager.vi"("error in"=w484, "glyph manager"=w475, "depth"=0 ("Depth"), "node self ref"=w482) -> ("error out"=w483:errorcluster, "glyph manager out"=w474:T9, "summary"=w470:T18[])  [unwired: 5 in]
        n173 = Index Array(array=w470) -> (element=w469:T18)  [unwired: 1 in]
        n174 = control-ref of="This VI"() -> (w485:refnum<vi>)
        n175 = Unbundle By Name(w469) -> ("ID"=w468:string)
        n176 = call <vilib>:"RefreshEntireTreeWithGlyphManager.vi"("calling VI in"=w485, "error in"=w483, "glyph manager"=w474, "array"=w470, "tree ref in"=w473) -> ("error out"=w479:errorcluster, "glyph manager out"=w476:T9)  [unwired: 5 in]
        n177 = control-ref of="Sub Panel"() -> (w480:refnum<vi>)
        n178 = call <vilib>:"ClearSubPanelStandardEvents.vi"("error in"=w479, "standard events"=w478, "sub panel ref in"=w480) -> ("error out"=w472:errorcluster)  [unwired: 7 in, 1 out]
        n179 = Bundle By Name(cluster=w486, "glyph manager"=w476) -> (w477:T1)
        n180 = disable-structure shown="Enabled" {
          disable-tunnel: w473 -> [w489 w493]
          disable-tunnel: w472 -> [w488 w495]
          disable-tunnel: [w487 w494] -> w471
          disable-tunnel: w468 -> [_ w492]
          disable-tunnel: w465 -> [_ w491]
          frame Disabled {
            # "#Change - Condense tree"
            n181 = invoke class="Tree (strict)" method="Open/Close.Open/Close All"(reference=w489, error in=w488, "Open"=FALSE ("Open?")) -> (error out=w487:errorcluster)  [unwired: 1 in, 3 out]
          }
          frame Enabled {
            n182 = case shown="True" w491 {
              tunnel: w495 -> [w496 w500]
              tunnel: [w496 w499] -> w494
              tunnel: w493 -> [_ w498]
              tunnel: w492 -> [_ w497]
              frame False {
              }
              frame True {
                n183 = property class="Tree (strict)"(reference=w498, error in=w500, "Val(Sgnl)"=w497) -> (error out=w499:errorcluster)  [unwired: 1 out]
              }
            }
          }
        }
      }
      frame "CleansubPanel" {
        n184 = Unbundle By Name(w505) -> ("standard events"=w501:T3)
        n185 = control-ref of="Sub Panel"() -> (w507:refnum<vi>)
        n186 = call <vilib>:"ClearSubPanelStandardEvents.vi"("error in"=w506, "standard events"=w501, "sub panel ref in"=w507) -> ("error out"=w504:errorcluster, "sub panel ref out"=w503:refnum<vi>)  [unwired: 7 in]
        n187 = Close Reference(reference=w503, error in (no error)=w504) -> (error out=w502:errorcluster)
      }
      frame "ActivateNode" {
        n188 = Unbundle By Name(w510) -> ("standard events"=w509:T3)
        n189 = call <vilib>:"IDtoNode.vi"("error in"=w515, "ID"=w516) -> ("error out"=w508:errorcluster, "invalid Id"=w514:bool, "node ref"=w513:T2)  [unwired: 7 in]
        n190 = case shown="False" w514 {
          tunnel: w513 -> [w523 _]
          tunnel: [w524 w525] -> w512
          tunnel: w508 -> [w521 w525]
          tunnel: w511 -> [w519 _]
          tunnel: w509 -> [w517 _]
          frame False {
            n191 = control-ref of="Sub Panel"() -> (w520:refnum<vi>)
            n192 = call <vilib>:"ClearSubPanelStandardEvents.vi"("error in"=w521, "standard events"=w517, "sub panel ref in"=w520) -> ("error out"=w522:errorcluster, "sub panel ref out"=w518:refnum<vi>)  [unwired: 7 in]
            n193 = call <vilib>:"LoadNodeUIStandardEvents.vi"("user event out"=w517, "error in"=w522, "sub panel ref in"=w518, "main queue"=w519, "node"=w523) -> ("error out"=w524:errorcluster)  [unwired: 6 in]
          }
          frame True {
          }
        }
      }
      frame "Move" {
        n194 = Unflatten From String(type=T14 {"node ref"=refnum, "new parent"=refnum} ("Cluster"), binary string=w536, error in (no error)=w534) -> (value=w533:T14, error out=w532:errorcluster)  [unwired: 2 in, 1 out]
        n195 = Unbundle By Name(w533) -> ("node ref"=w527:T2, "new parent"=w526:T2)
        n196 = call <vilib>:"MoveNode.vi"("error in"=w532, "new parent"=w526, "node"=w527) -> ("error out"=w530:errorcluster)  [unwired: 8 in]
        n197 = call <vilib>:"Send Local Message.vi"("message queue in"=w528, "message name"="PopulateTree", "error in"=w530) -> ("error out"=w529:errorcluster)  [unwired: 10 in, 2 out]
      }
      frame "NodeDataChange" {
        n198 = call <vilib>:"Send Local Message.vi"("message queue in"=w541, "message name"="RefreshNode", "message value"=w543, "error in"=w544) -> ("error out"=w542:errorcluster)  [unwired: 9 in, 2 out]
        n199 = Bundle By Name(cluster=w545, "unsaved changes"=TRUE) -> (w539:T1)
      }
    }
  }
  n200 = while "User Interface Event Handler" {
    tunnel: w21 -> [w554]
    tunnel: w20 -> [w550]
    tunnel: w13 -> [w549]
    tunnel: [w548] -> w9
    shift-right: [w546] -> _
    shift-left: w5 -> [w547]
    stop <- w553 stop-if-true
    n201 = event shown="[10] Panel Close?" {
      selector: w549 -> [_ _ _ _ _ _ _ _ _ _ _ _ _]
      dyn-events: [_ _ _ _ _ _ _ _ _ _ _ _ _] -> w548
      timeout: 1000 -> [_ _ _ _ _ _ _ _ _ _ _ _ _]
      tunnel: w554 -> [w558 w567 w592 w639 w646 w674 w703 w711 w741 w746 w757 w764 w811]
      tunnel: [_ _ _ _ _ _ TRUE _ _ _ _ _ _] -> w553
      tunnel: [w558 w567 w591 w639 w646 w672 w699 w711 w738 w746 w755 w763 w812] -> w552
      tunnel: [w557 w563 w590 _ w640 w671 w700 w707 w737 w743 w753 w761 _] -> w551
      tunnel: w550 -> [w557 w566 w589 _ w641 w673 w701 w710 w736 w745 w754 w762 _]
      tunnel: w547 -> [w556 w559 w585 w637 w642 w658 w698 w706 w735 w742 w752 w759 w809]
      tunnel: [w556 w559 w585 w637 w643 w658 w698 w706 w735 w742 w752 w759 w809] -> w546
      event Timeout {
        # "Timeout code can be added here for autosave or Lock Screen"
        n202 = event-data() -> ()  [unwired: 1 in, 1 out]
      }
      event "View": Shortcut Menu Activation? {
        n203 = event-data() -> ("CtlRef"=w573:refnum<vi>, "Coords"=w572:T19, "MenuRef"=w569:refnum<k9>)  [unwired: 1 in]
        n204 = invoke class="Tree (strict)" method="Point To Row Column"(reference=w573, error in=w566, "Point"=w572) -> (error out=w565:errorcluster, "Tag"=w571:string)  [unwired: 5 in, 6 out]
        n205 = call <vilib>:"IDtoNode.vi"("error in"=w565, "ID"=w571) -> ("error out"=w561:errorcluster, "invalid Id"=w568:bool, "node ref"=w570:T2)  [unwired: 7 in]
        n206 = case shown="False" w568 {
          tunnel: w570 -> [w578 _]
          tunnel: w569 -> [w577 _]
          tunnel: [w576 _] -> w564
          tunnel: [w575 _] -> w562
          tunnel: w561 -> [w574 w584]
          tunnel: [w574 w584] -> w560
          frame False {
            n207 = in-place {
              in-place-border: w577 -> [w581]
              in-place-border: [w579] -> w576
              n208 = in-place-dvr #8(w578) -> (w583:refnum<class "NISE_CEF_Node.lvclass">, w580:errorcluster)
              n209 = call-dynamic "ShortcutMenu.vi"("error in"=w580, "menu ref in"=w581, "node in"=w583) -> ("error out"=w579:errorcluster, "node out"=w582:refnum<class "NISE_CEF_Node.lvclass">)  [unwired: 6 in, 1 out]
              n210 = in-place-dvr #8(w582) -> (w575:errorcluster)  [unwired: 1 out]
            }
          }
          frame True {
          }
        }
        n211 = Merge Errors(w562, w564, w560) -> (w563:errorcluster)
        n212 = event-data() -> ()  [unwired: 2 in, 1 out]
      }
      event "View": Shortcut Menu Selection (User) {
        n213 = event-data() -> ("ItemPath"=w586:string, "CtlRef"=w595:refnum<vi>, "Coords"=w596:T19)  [unwired: 1 in]
        n214 = invoke class="Tree (strict)" method="Point To Row Column"(reference=w595, error in=w589, "Point"=w596) -> (error out=w588:errorcluster, "Tag"=w587:string)  [unwired: 5 in, 6 out]
        n215 = Match Pattern(string=w586, regular expression=":") -> (before substring=w594:string, after substring=w593:string)  [unwired: 1 in, 2 out]
        n216 = case shown="\"Add\"" w594 {
          selector: w594 -> [w598 _ _ _ _]
          tunnel: w593 -> [_ _ _ w622 w626]
          tunnel: w592 -> [w605 w612 w618 w624 w633]
          tunnel: w587 -> [w600 w610 w616 w621 w632]
          tunnel: [w602 w609 w615 w620 w630] -> w591
          tunnel: [w603 w608 w613 w619 w628] -> w590
          tunnel: w588 -> [w604 w607 w614 w623 w629]
          frame Default {
            n217 = Concatenate Strings(w598, ":" ("string"), w600) -> (w601:string)
            n218 = call <vilib>:"Send Local Message.vi"("message queue in"=w605, "message name"="CustomMenuAction" ("Message Name"), "message value"=w601, "error in"=w604) -> ("message queue out"=w602:T12, "error out"=w603:errorcluster)  [unwired: 9 in, 1 out]
          }
          frame "Remove" {
            n219 = call <vilib>:"Send Local Message.vi"("message queue in"=w612, "message name"="RemoveNode" ("Message Name"), "message value"=w610, "error in"=w607) -> ("message queue out"=w609:T12, "error out"=w608:errorcluster)  [unwired: 9 in, 1 out]
          }
          frame "Duplicate" {
            n220 = call <vilib>:"Send Local Message.vi"("message queue in"=w618, "message name"="Duplicate" ("Message Name"), "message value"=w616, "error in"=w614) -> ("message queue out"=w615:T12, "error out"=w613:errorcluster)  [unwired: 9 in, 1 out]
          }
          frame "Add" {
            n221 = call "Send Message to Create Child Object.vi"("Error In"=w623, "ID of Node to Add To"=w621, "node type"=w622, "Queue in"=w624) -> ("Error Out"=w619:errorcluster, "Queue Out"=w620:T12)  [unwired: 6 in]
          }
          frame "New" {
            n222 = Match Pattern(string=w626, regular expression=":") -> (after substring=w625:string)  [unwired: 1 in, 3 out]
            n223 = Bundle By Name(cluster=T13 {"node type"="", "to add to"=""} ("input cluster"), "node type"=w625, "to add to"=w632) -> (w634:T13)
            n224 = Flatten To String(anything=w634) -> (data string=w635:string)  [unwired: 3 in, 2 out]
            n225 = call <vilib>:"Send Local Message.vi"("message queue in"=w633, "message name"="AddNode" ("Message Name"), "message value"=w635, "error in"=w629) -> ("message queue out"=w630:T12, "error out"=w628:errorcluster)  [unwired: 9 in, 1 out]
          }
        }
      }
      event "VeriStand Version": Value Change {
        n226 = event-data() -> ()  [unwired: 1 in, 6 out]
        n227 = global write "Global Settings.vi" "VeriStand Version"("VeriStand Version") -> ()
      }
      event "Target Project": Value Change {
        n228 = event-data() -> ("OldVal"=w644:string)  [unwired: 1 in, 5 out]
        n229 = case shown="Default" "Target Project" {
          selector: "Target Project" -> [_ w656]
          tunnel: w644 -> [w651 _]
          tunnel: [w649 w655] -> w643
          tunnel: w642 -> [_ w655]
          tunnel: w641 -> [w648 w654]
          tunnel: [w647 w653] -> w640
          frame "Refresh..." {
            n230 = control-ref of="Target Project"() -> (w652:refnum<vi>)
            n231 = call "Initialize Target Project.vi"("error in (no error)"=w648, "ComboBox in"=w652) -> ("error out"=w650:errorcluster, "Projects"=w649:T11)  [unwired: 8 in]
            n232 = call "Set Target Project.vi"("error in (no error)"=w650, "Target Project"=w651, "Projects"=w649, "ComboBox Ref"=w652) -> ("error out"=w647:errorcluster)  [unwired: 7 in]
          }
          frame Default {
            n233 = control-ref of="Target Project"() -> (w657:refnum<vi>)
            n234 = call "Set Target Project.vi"("error in (no error)"=w654, "Target Project"=w656, "Projects"=w655, "ComboBox Ref"=w657) -> ("error out"=w653:errorcluster)  [unwired: 7 in]
          }
        }
      }
      event "View": Drop {
        n235 = event-data() -> ("CtlRef"=w677:refnum<vi>, "Coords"=w676:T19)  [unwired: 1 in]
        n236 = invoke class="Tree (strict)" method="Point To Row Column"(reference=w677, error in=w673, "Point"=w676) -> (reference out=w675:refnum<vi>, error out=w670:errorcluster, "Tag"=w667:string)  [unwired: 5 in, 5 out]
        n237 = call <vilib>:"ValidDragDrop.vi"("error in"=w670, "drag over"=w667, "Tree Ref in"=w675) -> ("Error Out"=w662:errorcluster, "Accepted"=w665:bool, "Drag"=w669:string, "Tree Ref out"=w679:refnum<vi>)  [unwired: 1 in, 4 out]
        n238 = call <vilib>:"IDtoNode.vi"("error in"=w662, "ID"=w667) -> ("error out"=w663:errorcluster, "invalid Id"=w660:bool, "node ref"=w666:T2)  [unwired: 7 in]
        n239 = call <vilib>:"IDtoNode.vi"("error in"=w663, "ID"=w669) -> ("error out"=w661:errorcluster, "invalid Id"=w659:bool, "node ref"=w668:T2)  [unwired: 7 in]
        n240 = Compound Arithmetic op=AND(w665, invert w660, invert w659) -> (w664:bool)
        n241 = case shown="True" w664 {
          tunnel: w669 -> [_ w695]
          tunnel: w679 -> [_ w697]
          tunnel: [_ TRUE] -> w678
          tunnel: w667 -> [_ w693]
          tunnel: w674 -> [w681 w692]
          tunnel: [w681 w688] -> w672
          tunnel: [w680 w687] -> w671
          tunnel: w668 -> [_ w683]
          tunnel: w666 -> [_ w682]
          tunnel: w661 -> [w680 w684]
          frame False {
          }
          frame True {
            n242 = invoke class="Tree (strict)" method="Edit Tree Items.Move Item"(reference=w697, error in=w684, "tag"=w695, "New Parent"=w693) -> (error out=w685:errorcluster)  [unwired: 3 in, 6 out]
            n243 = Bundle By Name(cluster=T14 {"node ref"=refnum, "new parent"=refnum} ("Cluster"), "new parent"=w682, "node ref"=w683) -> (w691:T14)
            n244 = Flatten To String(anything=w691, error in (no error)=w685) -> (data string=w690:string, error out=w686:errorcluster)  [unwired: 2 in, 1 out]
            n245 = call <vilib>:"Send Local Message.vi"("message queue in"=w692, "message name"="Move", "message value"=w690, "error in"=w686) -> ("message queue out"=w688:T12, "error out"=w687:errorcluster)  [unwired: 9 in, 1 out]
          }
        }
        n246 = event-data("Accepted?"=w678) -> ()  [unwired: 1 in, 1 out]
      }
      event "Exit": Value Change {
        # "Exit the application                                           >> Stop this message generator loop    Cleaning errors if the other loop stop this one"
        n247 = event-data() -> ()  [unwired: 1 in, 1 out]
        n248 = call <vilib>:"Send Local Message.vi"("message queue in"=w703, "message name"="Close", "error in"=w701) -> ("message queue out"=w699:T12, "error out"=w704:errorcluster)  [unwired: 10 in, 1 out]
        n249 = call <vilib>:"Clear Errors.vi"("error in (no error)"=w704) -> ("error out"=w700:errorcluster)  [unwired: 5 in, 1 out]
      }
      event "View": Drag Starting? {
        n250 = event-data() -> ("Data"=w717:T20, "CtlRef"=w719:refnum<vi>, "Coords"=w718:T19)  [unwired: 1 in]
        n251 = invoke class="Tree (strict)" method="Point To Row Column"(reference=w719, error in=w710, "Point"=w718) -> (error out=w709:errorcluster, "Tag"=w716:string)  [unwired: 5 in, 6 out]
        n252 = call <vilib>:"IDtoNode.vi"("error in"=w709, "ID"=w716) -> ("error out"=w708:errorcluster, "invalid Id"=w715:bool, "node ref"=w714:T2)  [unwired: 7 in]
        n253 = case shown="False" w715 {
          tunnel: w714 -> [w727 _]
          tunnel: [w724 TRUE ("Removable")] -> w712
          tunnel: w708 -> [w723 w733]
          tunnel: [w720 w733] -> w707
          frame False {
            n254 = in-place {
              in-place-border: [w730] -> w726
              in-place-border: w723 -> [w729]
              in-place-border: [w728] -> w722
              n255 = in-place-dvr #9(w727) -> (w732:refnum<class "NISE_CEF_Node.lvclass">)  [unwired: 1 out]
              n256 = call-dynamic "EditOptions.vi"("error in"=w729, "node in"=w732) -> ("error out"=w728:errorcluster, "edit options"=w730:T21, "node out"=w731:refnum<class "NISE_CEF_Node.lvclass">)  [unwired: 6 in, 1 out]
              n257 = in-place-dvr #9(w731) -> (w721:errorcluster)  [unwired: 1 out]
            }
            n258 = Unbundle By Name(w726) -> ("movable"=w725:bool)
            n259 = Merge Errors(w721, w722) -> (w720:errorcluster)
            n260 = Not(x=w725) -> (.not. x?=w724:bool)
          }
          frame True {
          }
        }
        n261 = event-data("Data"=w717, "Drag Mode"=enum32{"copy or move", "copy only", "move only"}."move only", "Discard?"=w712) -> ()  [unwired: 1 in, 1 out]
      }
      event "View": Value Change {
        n262 = event-data() -> ("NewVal"=w739:string)  [unwired: 1 in]
        n263 = call <vilib>:"Send Local Message.vi"("message queue in"=w741, "message name"="ActivateNode" ("Message Name"), "message value"=w739, "error in"=w736) -> ("message queue out"=w738:T12, "error out"=w737:errorcluster)  [unwired: 9 in, 1 out]
      }
      event "View": event type 3.0.xa000003a {
        n264 = event-data() -> ("CtlRef"=w751:refnum<vi>, "Coords"=w748:T19)  [unwired: 1 in]
        n265 = invoke class="Tree (strict)" method="Point To Row Column"(reference=w751, error in=w745, "Point"=w748) -> (reference out=w750:refnum<vi>, error out=w744:errorcluster, "Tag"=w749:string)  [unwired: 5 in, 5 out]
        n266 = call <vilib>:"ValidDragDrop.vi"("error in"=w744, "drag over"=w749, "Tree Ref in"=w750) -> ("Error Out"=w743:errorcluster, "Accepted"=w747:bool)  [unwired: 1 in, 6 out]
        n267 = event-data("Accepted?"=w747) -> ()  [unwired: 1 in, 1 out]
      }
      event Panel Close? {
        # "Intercepts the upper right close panel operation to allow a smooth shutdown as opposed to immediately killing the app."
        n268 = event-data() -> ()  [unwired: 1 in, 1 out]
        n269 = call <vilib>:"Send Local Message.vi"("message queue in"=w757, "message name"="Close?", "error in"=w754) -> ("message queue out"=w755:T12, "error out"=w753:errorcluster)  [unwired: 10 in, 1 out]
        n270 = event-data("Discard?"=TRUE) -> ()  [unwired: 1 in, 1 out]
      }
      event Menu Selection (User) {
        # "#USERCFG It is needed to add a Case for Every item on the menu"
        n271 = event-data() -> ("ItemTag"=w760:string, "ItemPath"=w765:string)  [unwired: 1 in]
        n272 = case shown="Default" w765 {
          selector: w765 -> [w769 _ _ _ _ _ _]
          tunnel: w764 -> [w774 w779 w784 w789 w794 w799 w808]
          tunnel: [w774 w775 w780 w785 w790 w795 w805] -> w763
          tunnel: w762 -> [w771 w777 w782 w787 w792 w797 w804]
          tunnel: [w770 w776 w781 w786 w791 w796 w802] -> w761
          tunnel: w760 -> [w768 _ _ _ _ _ _]
          frame Default {
            n273 = Concatenate Strings(w768, "::" ("string"), w769) -> (w767:string)
            n274 = call <vilib>:"NISE_error generator.vi"("error in"=w771, "source"="configuration tool main.vi", "append error message"=w767, "error code (0)"=538506) -> ("error out"=w770:errorcluster)  [unwired: 5 in]
          }
          frame "_File:_New" {
            n275 = call <vilib>:"Send Local Message.vi"("message queue in"=w779, "message name"="New?" ("Message Name"), "error in"=w777) -> ("message queue out"=w775:T12, "error out"=w776:errorcluster)  [unwired: 10 in, 1 out]
          }
          frame "_File:_Open" {
            n276 = call <vilib>:"Send Local Message.vi"("message queue in"=w784, "message name"="Open?" ("Message Name"), "error in"=w782) -> ("message queue out"=w780:T12, "error out"=w781:errorcluster)  [unwired: 10 in, 1 out]
          }
          frame "_File:_Save" {
            n277 = call <vilib>:"Send Local Message.vi"("message queue in"=w789, "message name"="Save" ("Message Name"), "error in"=w787) -> ("message queue out"=w785:T12, "error out"=w786:errorcluster)  [unwired: 10 in, 1 out]
          }
          frame "_File:Save As..." {
            n278 = call <vilib>:"Send Local Message.vi"("message queue in"=w794, "message name"="SaveAs" ("Message Name"), "error in"=w792) -> ("message queue out"=w790:T12, "error out"=w791:errorcluster)  [unwired: 10 in, 1 out]
          }
          frame "_File:_Exit" {
            n279 = call <vilib>:"Send Local Message.vi"("message queue in"=w799, "message name"="Close?" ("Message Name"), "error in"=w797) -> ("message queue out"=w795:T12, "error out"=w796:errorcluster)  [unwired: 10 in, 1 out]
          }
          frame "_Tools:Multiple Parameter Editor" {
            n280 = call <vilib>:"Send Local Message.vi"("message queue in"=w808, "message name"="CleansubPanel", "error in"=w804) -> ("message queue out"=w807:T12, "error out"=w803:errorcluster)  [unwired: 10 in, 1 out]
            n281 = call <vilib>:"Send Local Message.vi"("message queue in"=w807, "message name"="Custom View" ("Message Name"), "message value"="Multiple Variable Editor" ("Message Name"), "error in"=w803) -> ("message queue out"=w805:T12, "error out"=w802:errorcluster)  [unwired: 9 in, 1 out]
          }
        }
      }
      event User Event {
        n282 = event-data() -> ("node ref"=w810:T2)  [unwired: 1 in]
        n283 = call <vilib>:"NodetoID.vi"("node ref"=w810) -> ("ID"=w813:string)  [unwired: 9 in, 1 out]
        n284 = call <vilib>:"Send Local Message.vi"("message queue in"=w811, "message name"="NodeDataChange", "message value"=w813) -> ("message queue out"=w812:T12)  [unwired: 10 in, 2 out]
      }
    }
    n285 = call "Error.vi"("error in (no error)"=w551, "message queue in"=w552) -> ()  [unwired: 9 in, 1 out]
  }
  n286 = Unregister For Events(event registration refnum=w9) -> (error out=w10:errorcluster)  [unwired: 1 in]
  n287 = Merge Errors(w10, w15) -> (w11:errorcluster)
  n288 = call <vilib>:"DestroyStandardEvents.vi"("error in"=w11, "standard events"=w14) -> ()  [unwired: 9 in, 1 out]
